vi "peak - phase around center.vi"(8 "4corners":T1={"z (-pi/2)"=-1.0311345636926572+0.5736824521422934i, "z(inf)"=-0.5200164984937075+1.0975277942502903i, "z (pi/2)"=-1.0311345636926572+0.5736824521422934i, "z center"=-0.5136528600391839+0.580046090596817i, "z(0)"=-0.5200164984937075+1.0975277942502903i, "radius"=-1.0311345636926572}, 11 "z":cdb[](array[numeric])) -> (2 "Unwrapped Phase":dbl[](array[numeric]))   [LabVIEW 2017]
uses:
  circle corners.ctl
  <vilib>/Analysis/NI_AALPro.lvlib
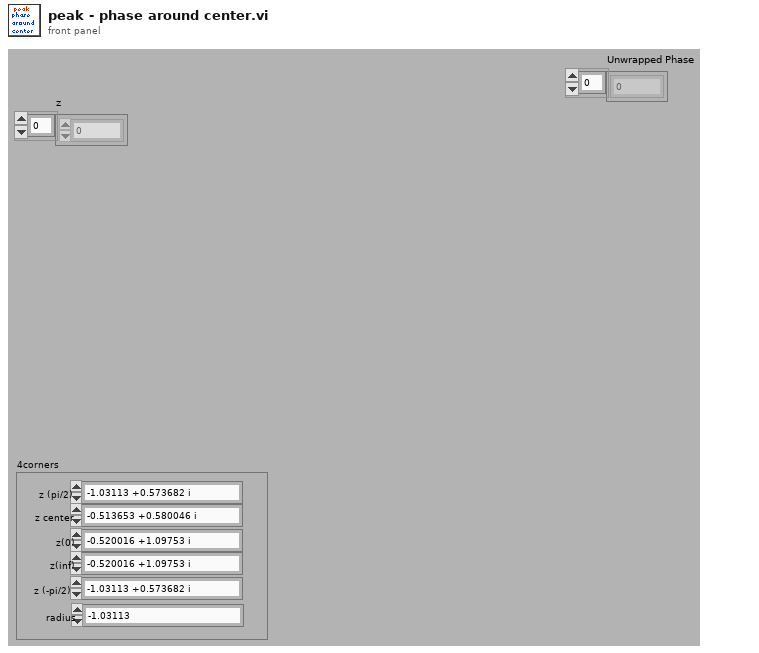
[diagram p1: front panel]
types:
  T1 = typedef "circle corners.ctl" = cluster{"z (-pi/2)":cdb, "z(inf)":cdb, "z (pi/2)":cdb, "z center":cdb, "z(0)":cdb, "radius":dbl}
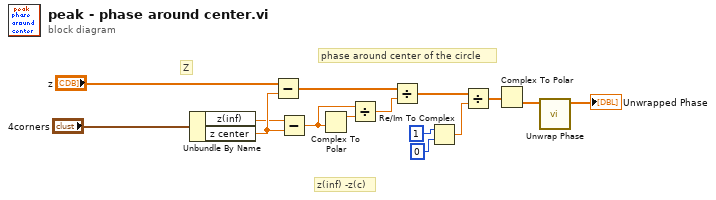
[diagram p0: block diagram]
diagram:
  # "Z"
  # "phase around center of the circle"
  # "z(inf) -z(c)"
  n1 = Unbundle By Name("4corners") -> ("z(inf)"=w2:cdb, "z center"=w3:cdb)
  n2 = Subtract(x="z", y=w3) -> (x-y=w11:cdb[])
  n3 = Subtract(x=w2, y=w3) -> (x-y=w1:cdb)
  n4 = Complex To Polar(r * e^(i*theta)=w1) -> (r=w12:dbl)  [unwired: 1 out]
  n5 = Divide(x=w1, y=w12) -> (x/y=w4:cdb)
  n6 = Divide(x=w11, y=w4) -> (x/y=w7:cdb[])
  n7 = Re/Im To Complex(1:0, 2:1) -> (0:w9:cdb)
  n8 = Divide(x=w7, y=w9) -> (x/y=w10:cdb[])
  n9 = Complex To Polar(r * e^(i*theta)=w10) -> (theta=w5:dbl[])  [unwired: 1 out]
  n10 = call <vilib>:"Unwrap Phase.vi"("Phase"=w5) -> ("Unwrapped Phase"=→"Unwrapped Phase":dbl[])  [unwired: 9 in, 1 out]
